vi "write-read placa.vi"(0 "Write Command":string, 2 "COM DATA":T1={"IP "="192.168.1.7", "Puerto:"=2101, "Time Out"=500}, 3 "bytes":u16) -> (5 "LECTURA":string, 6 "COM FAIL":bool caption="COM\nFAIL", 7 "error out":errorcluster)   [LabVIEW 2010]
uses:
  <vilib>/regexp/Match Regular Expression.xnode
panel:
  out "error out 2":errorcluster
  out "bytes DEL":i32
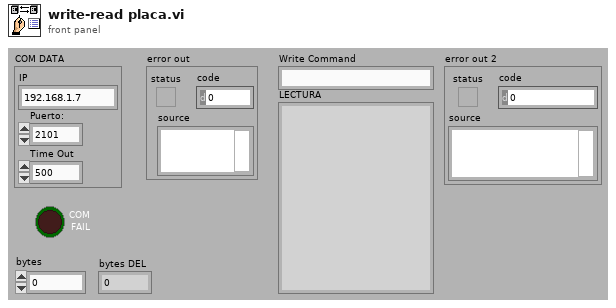
[diagram p1: front panel]
types:
  T1 = cluster{"IP ":string, "Puerto:":u16, "Time Out":u16}
  T2 = cluster{"connection ID":refnum<k5>, "Time Out":u16, "error out":errorcluster}
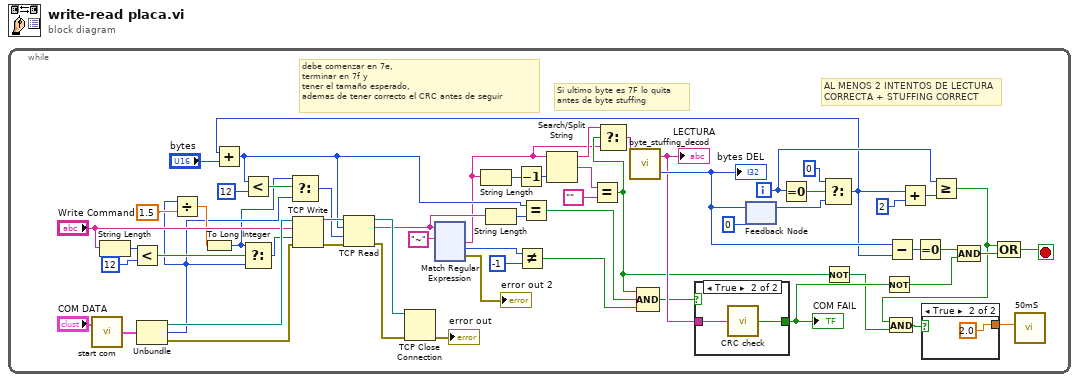
[diagram p0: block diagram]
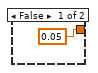
[diagram p2: hidden frame]
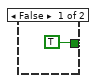
[diagram p3: hidden frame]
diagram:
  n1 = while {
    i -> [w25]
    stop <- w10 stop-if-true
    # "Si ultimo byte es 7F lo quita\nantes de byte stuffing"
    # "debe comenzar en 7e,\nterminar en 7f y\ntener el tamaño esperado, \nademas de tener correcto el CRC antes de seguir"
    # "AL MENOS 2 INTENTOS DE LECTURA\nCORRECTA + STUFFING CORRECT"
    n2 = call "start com.vi"("COM DATA"="COM DATA") -> ("ONLINE OUT"=w36:T2)  [unwired: 1 in]
    n3 = String Length(string="Write Command") -> (length=w22:i32)
    n4 = Less?(x=w22, y=12) -> (x < y?=w20:bool)
    n5 = Unbundle(w36) -> ("connection ID"=w34:refnum<k5>, "Time Out"=w12:u16, "error out"=w33:errorcluster)
    n6 = Divide(x=w12, y=1.5) -> (x/y=w17:dbl)
    n7 = To Long Integer(number=w17) -> (32bit integer=w11:i32)
    n8 = Select(t=w11, s=w20, f=w12) -> (s? t:f=w19:i32)
    n9 = TCP Write(connection ID=w34, data in="Write Command", error in (no error)=w33, 9:w19) -> (connection ID out=w60:refnum<k5>, error out=w59:errorcluster)  [unwired: 1 out]
    n10 = feedback #1(0) -> (w28:i32)
    n11 = Equal To 0?(x=w25) -> (x = 0?=w30:bool)
    n12 = Select(t=0, s=w30, f=w28) -> (s? t:f=w24:i32)
    n13 = Add(x=w24, y="bytes") -> (x+y=w16:i32)
    n14 = Less?(x=w16, y=12) -> (x < y?=w14:bool)
    n15 = Select(t=w11, s=w14, f=w12) -> (s? t:f=w13:i32)
    n16 = TCP Read(connection ID=w60, bytes to read=w16, error in (no error)=w59, 9:w13) -> (connection ID out=w37:refnum<k5>, data out=w9:string, error out=w27:errorcluster)  [unwired: 1 in]
    n17 = TCP Close Connection(connection ID=w37, error in (no error)=w27) -> (error out=→"error out":errorcluster)  [unwired: 1 in, 1 out]
    n18 = xnode "Match Regular Expression"("input string"=w9, "regular expression"="~" ("Write Command 2")) -> ("after match"=w1:string, "offset past match"=w47:i32, "error out"=→"error out 2":errorcluster)  [unwired: 4 in, 2 out]
    n19 = String Length(string=w1) -> (length=w41:i32)
    n20 = String Length(string=w9) -> (length=w54:i32)
    n21 = Decrement(x=w41) -> (x-1=w42:i32)
    n22 = Not Equal?(x=w47, y=-1) -> (x != y?=w53:bool)
    n23 = Equal?(x=w16, y=w54) -> (x = y?=w52:bool)
    n24 = Search/Split String(string=w1, offset (0)=w42) -> (substring before match=w2:string, match + rest of string=w40:string)  [unwired: 1 in, 1 out]
    n25 = Equal?(x=w40, y="" ("Write Command 2")) -> (x = y?=w3:bool)
    n26 = Select(t=w2, s=w3, f=w1) -> (s? t:f=w4:string)
    n27 = call "byte_stuffing_decod.vi"("String IN"=w4) -> ("bytes DEL"=w48:i32, "String OUT"=w44:string)  [unwired: 1 in]
    "LECTURA" <- w44
    "bytes DEL" <- w48
    n28 = Compound Arithmetic op=AND(w3, w52, w53) -> (w43:bool)
    n29 = case shown="True" w43 {
      tunnel: w44 -> [_ w65]
      tunnel: [TRUE ("CRC fail") w64] -> w32
      frame False {
      }
      frame True {
        n30 = call "CRC check.vi"("data IN"=w65) -> ("CRC fail"=w64:bool)
      }
    }
    "COM FAIL" <- w32
    n31 = feedback-in #1(w48) -> ()
    n32 = Not(x=w3) -> (.not. x?=w6:bool)
    n33 = Not(x=w32) -> (.not. x?=w31:bool)
    n34 = Subtract(x=w48, y=w24) -> (x-y=w50:i32)
    n35 = Add(x=w24, y=2) -> (x+y=w55:i32)
    n36 = Equal To 0?(x=w50) -> (x = 0?=w45:bool)
    n37 = Greater Or Equal?(x=w25, y=w55) -> (x >= y?=w5:bool)
    n38 = And(x=w5, y=w6) -> (x .and. y?=w8:bool)
    n39 = case shown="True" w8 {
      tunnel: [0.05 ("Delay Time (s)") 2.0 ("Delay Time (s)")] -> w7
      frame False {
      }
      frame True {
      }
    }
    n40 = Compound Arithmetic op=AND(w45, w31) -> (w46:bool)
    n41 = Compound Arithmetic op=OR(w5, w46) -> (w10:bool)
    n42 = call "50mS"("Delay Time (s)"=w7) -> ()  [unwired: 10 in, 1 out]
  }
